vi "create.vi"(5 "MultipartForm in":refnum<class "MultipartForm.lvclass">, 8 "error in (no error)":errorcluster) -> (0 "error out":errorcluster, 3 "MultipartForm out":refnum<class "MultipartForm.lvclass">)   [LabVIEW 2020, in "reqwest.lvlib" / "MultipartForm.lvclass"]
uses:
  MultipartForm.lvclass
  MultipartForm.lvclass/MultipartForm.ctl
  lv_reqwest_64.so
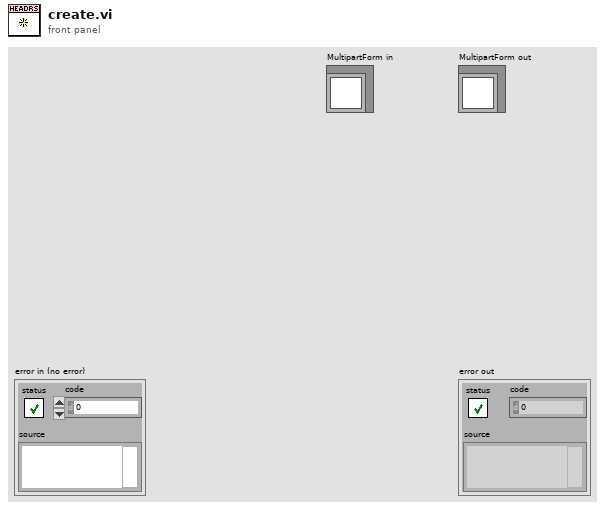
[diagram p1: front panel]
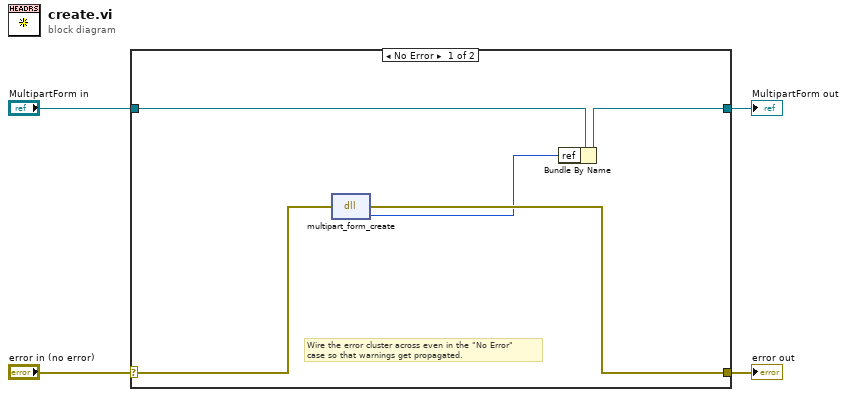
[diagram p0: block diagram]
diagram:
  n1 = case shown="No Error" "error in (no error)" {
    selector: "error in (no error)" -> [w8 w11]
    tunnel: [w7 w11] -> w3
    tunnel: [w6 w10] -> w1
    tunnel: "MultipartForm in" -> [w9 w10]
    frame No Error {
      # "Wire the error cluster across even in the \"No Error\"\ncase so that warnings get propagated."
      n2 = dll-call lib="home/jim-kring/Projects/reqwest-rs-labview/lv_src/lv_reqwest_*.*" fn="multipart_form_create"(error in=w8) -> (error out=w7:errorcluster, "value"=w5:u64)  [unwired: 2 in, 1 out]
      n3 = Bundle By Name(cluster=w9, "ref"=w5) -> (w6:refnum<class "MultipartForm.lvclass">)
    }
    frame Error {
    }
  }
  "error out" <- w3
  "MultipartForm out" <- w1
